vi "BallShear_PackageCapture.vi"(8 "Target Name":string, 9 "Capture":bool, 11 "Target Path":path) -> (0 "Success":bool, 3 "Actual Image Path":path)   [LabVIEW 2013]
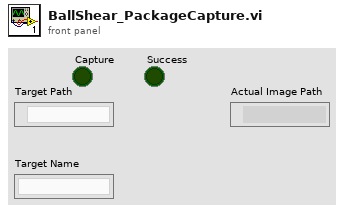
[diagram p1: front panel]
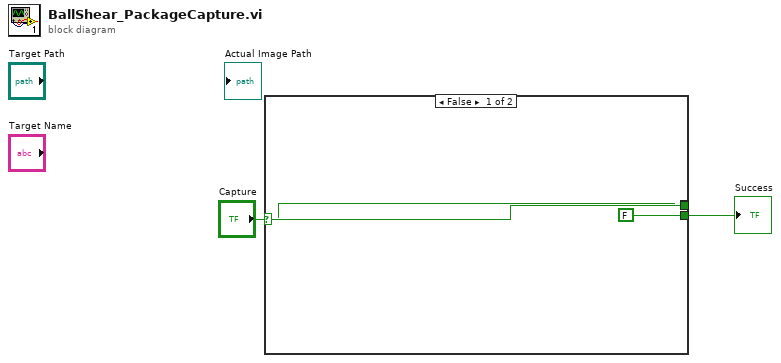
[diagram p0: block diagram]
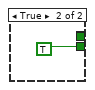
[diagram p2: hidden frame]
diagram:
  n1 = case shown="False" "Capture" {
    selector: "Capture" -> [w3 _]
    tunnel: [w3 w6] -> _
    tunnel: "Capture" -> [_ w6]
    tunnel: [FALSE ("Power") TRUE ("Power")] -> w1
    frame False {
    }
    frame True {
    }
  }
  "Success" <- w1
